vi "AddWeighted.vi"(6 "Gamma":i32, 7 "Alpha":sgl, 10 "Src2":u8[][](array[numeric]), 11 "Src1":u8[][](array[numeric])) -> (3 "Weighted Add":u8[][](array[numeric]))   [LabVIEW 2024]
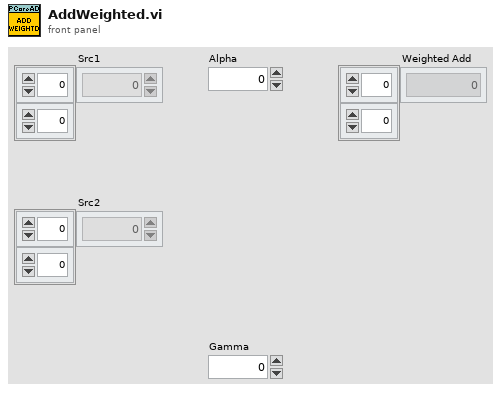
[diagram p1: front panel]
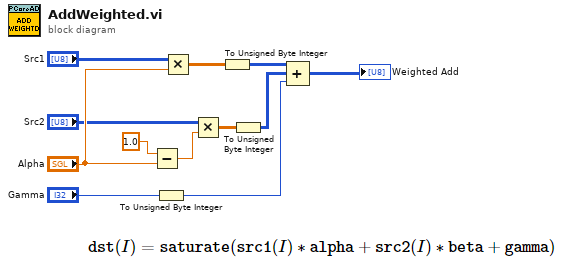
[diagram p0: block diagram]
diagram:
  n1 = Subtract(x=sgl 1.0, y="Alpha") -> (x-y=w10:sgl)
  n2 = To Unsigned Byte Integer(number="Gamma") -> (unsigned 8bit integer=w1:u8)
  n3 = Multiply(x="Src1", y="Alpha") -> (x*y=w7:sgl[][])
  n4 = Multiply(x="Src2", y=w10) -> (x*y=w4:sgl[][])
  n5 = To Unsigned Byte Integer(number=w7) -> (unsigned 8bit integer=w3:u8[][])
  n6 = To Unsigned Byte Integer(number=w4) -> (unsigned 8bit integer=w2:u8[][])
  n7 = Compound Arithmetic op=ADD(w3, w2, w1) -> (→"Weighted Add":u8[][])
